vi "testing3dgraph.vi"() -> ()   [LabVIEW 2017]
uses:
  <vilib>/Native 3D Graph/xcontrol/3DPC_SurfacePlot.xctl
  <vilib>/Utility/file.llb/Read Delimited Spreadsheet (DBL).vi
panel:
  in  "Select File to get \nAverage Trajectory":path=path "" caption="start path"
  out "3D Graph":refnum<class "Base Datatype.lvclass">[](xcontrol)
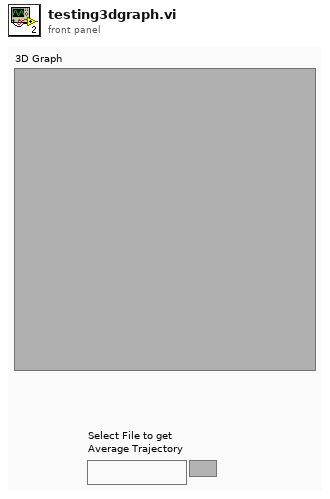
[diagram p1: front panel]
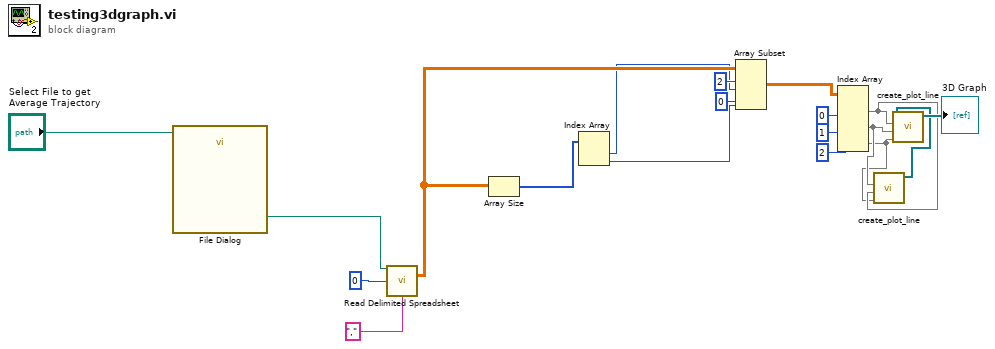
[diagram p0: block diagram]
diagram:
  n1 = call "File Dialog"("start path"="Select File to get \nAverage Trajectory") -> ("selected path"=w16:path)  [unwired: 11 in, 3 out]
  n2 = call-poly <vilib>:"Read Delimited Spreadsheet.vi"("file path (dialog if empty)"=w16, "start of read offset (chars.:0)"=0, "delimiter (\\t)"="," ("delimiter (\\t)")) -> ("all rows"=w13:dbl[][])  [unwired: 7 in, 5 out]
  n3 = Array Size(array=w13) -> (size(s)=w12:i32[])
  n4 = Index Array(array=w12) -> (element #1=w11:i32, element #2=w10:i32)  [unwired: 2 in]
  n5 = Array Subset(array=w13, index (row)=2 ("index"), length (row)=w11, index (col)=0 ("index"), length (col)=w10) -> (w9:dbl[][])
  n6 = Index Array(array=w9, index (col) #1=0 ("disabled index (col)"), index (col) #2=1 ("index (col)"), index (col) #3=2 ("index (col)")) -> (element #1=w2:dbl[], element #2=w3:dbl[], element #3=w1:dbl[])  [unwired: 3 in]
  n7 = call <vilib>:"create_plot_line.vi"("z vector"=w1, "y vector"=w2, "x vector"=w3) -> ("plots out"=w4:refnum<class "Base Datatype.lvclass">[])  [unwired: 2 in, 6 out]
  n8 = call <vilib>:"create_plot_line.vi"("z vector"=w1, "y vector"=w3, "x vector"=w2, "plots in"=w4) -> ("plots out"=→"3D Graph":refnum<class "Base Datatype.lvclass">[])  [unwired: 1 in, 6 out]
